vi "Node Example.vi"() -> ()   [LabVIEW 2016, in "PXImc Custom Device Engine.lvlib" / "PXImc Router.lvlib"]
uses:
  Shared/PXImc Router/Controls/Node - Configuration.ctl
  Shared/PXImc Router/Controls/Table Index-Size.ctl
  <vilib>/Utility/error.llb/DialogType.ctl
  Shared/PXImc Router/VIs/Node/Node - Globals.vi
  PXImc Router.lvlib
  Shared/PXImc Router/PXImc Router.lvlib
panel:
  in  "stop":bool
  out "Writer Node 2":T1(graph)={"[0]"=11.0, "[1]"=12.0, "[2]"=13.0, "[3]"=14.0, "[4]"=15.0, "[5]"=0.0, "[6]"=0.0, "[7]"=0.0, "[8]"=0.0}
  out "Writer Node 1":T1(graph)={"[0]"=1.0, "[1]"=2.0, "[2]"=3.0, "[3]"=4.0, "[4]"=5.0, "[5]"=0.0, "[6]"=0.0, "[7]"=0.0, "[8]"=0.0}
  out "Reader Node 2":T1(graph)
  out "Reader Node 1":T1(graph)
  in  "Node 2 Configuration Properties":T2={"Resource Name"="PXIMC2", "Node ID"=0, "Node Reader Conn Id"=4, "Node Writer Conn Id"=3, "Node # Channels"=5, "Writing Segments"={"Index"=5, "Size"=5}, "Reading Segments"={"Index"=0, "Size"=5}, "Connection Timeout (s)"=60.0, "Readers Buffer Size"=250000, "Slave IP Address"=""}
  in  "Node Configuration Properties":T2={"Resource Name"="PXIMC2", "Node ID"=0, "Node Reader Conn Id"=2, "Node Writer Conn Id"=1, "Node # Channels"=5, "Writing Segments"={"Index"=0, "Size"=5}, "Reading Segments"={"Index"=0, "Size"=5}, "Connection Timeout (s)"=60.0, "Readers Buffer Size"=250000, "Slave IP Address"=""}
  # "Node 1"
  # "Node 2"
  # "Node 2 => Node 1"
  # "Node 1 => Node 2"
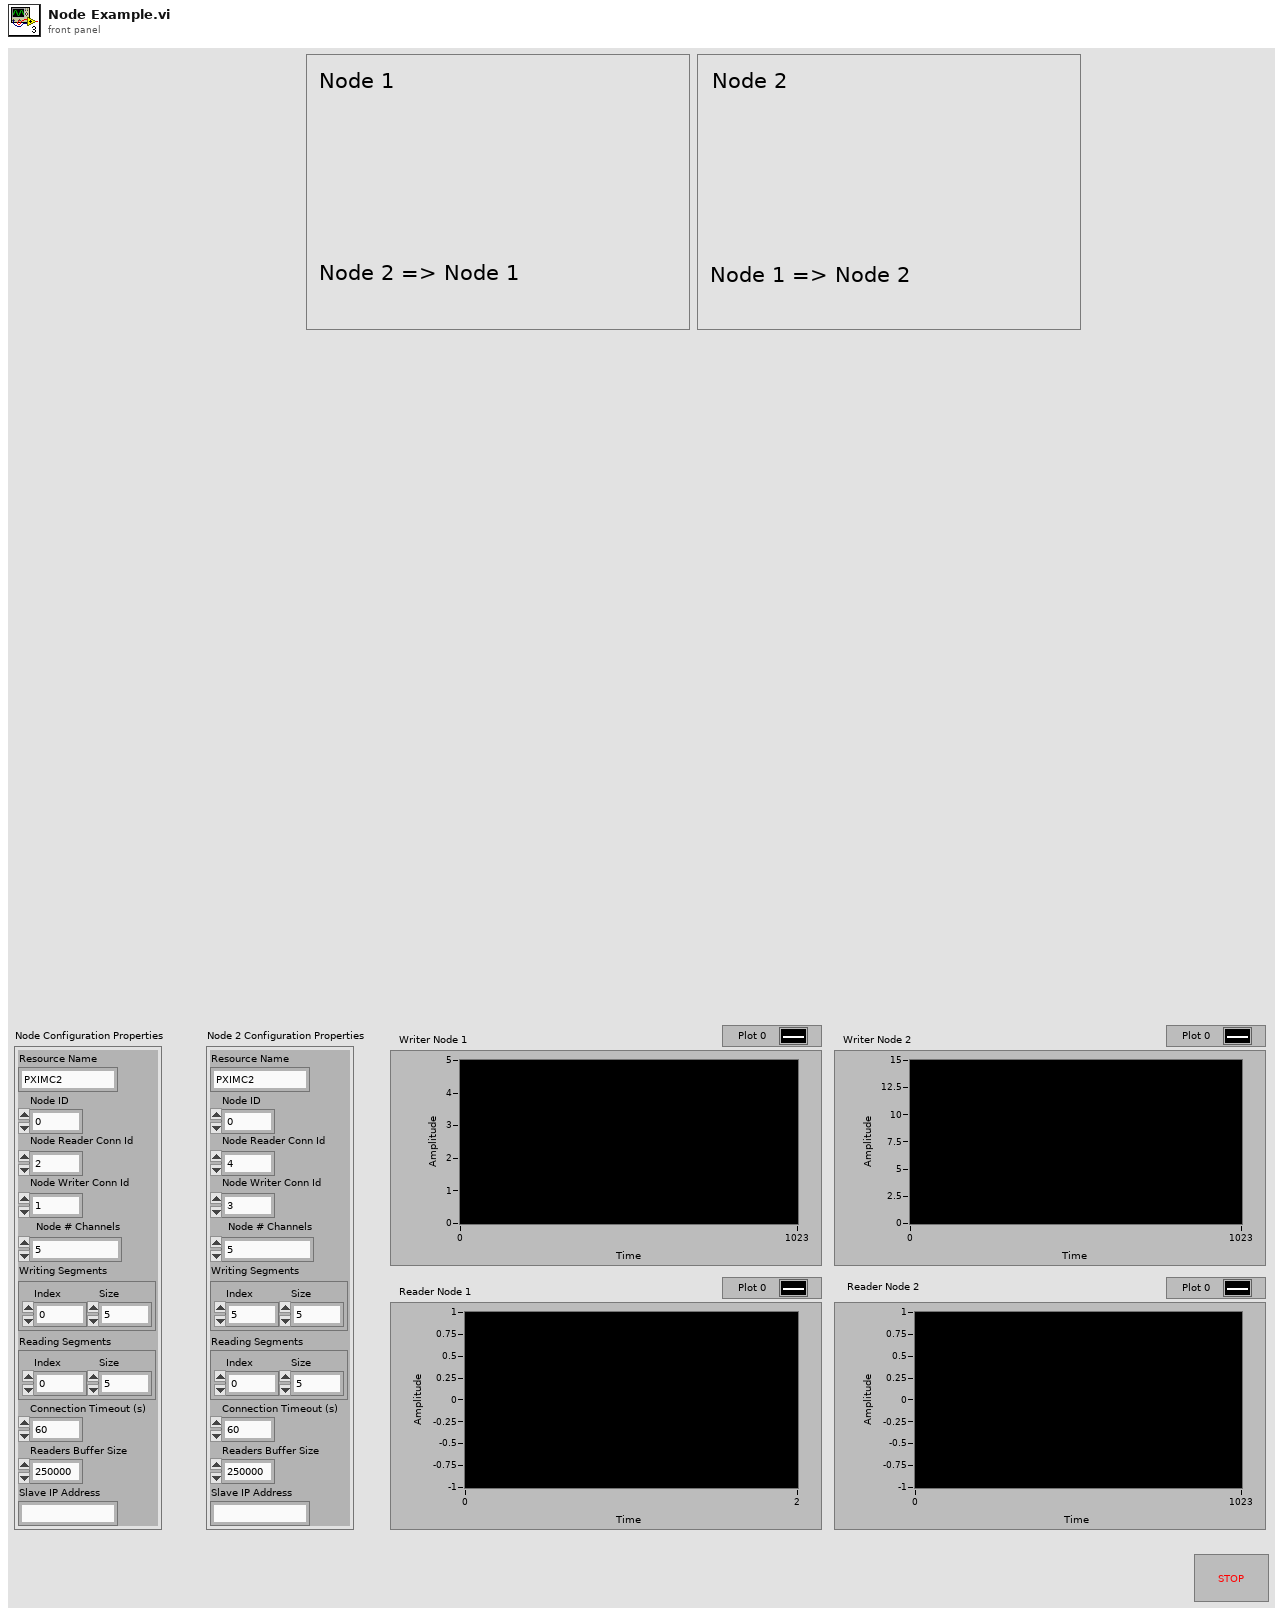
[diagram p1: front panel]
types:
  T1 = cluster{"[0]":dbl, "[1]":dbl, "[2]":dbl, "[3]":dbl, "[4]":dbl, "[5]":dbl, "[6]":dbl, "[7]":dbl, "[8]":dbl}
  T2 = typedef "PXImc Router.lvlib/Node - Configuration.ctl" = cluster{"Resource Name":string, "Node ID":u16, "Node Reader Conn Id":u16, "Node Writer Conn Id":u16, "Node # Channels":u32, "Writing Segments":T3, "Reading Segments":T3, "Connection Timeout (s)":dbl, "Readers Buffer Size":u32, "Slave IP Address":string}
  T3 = typedef "PXImc Router.lvlib/Table Index-Size.ctl" = cluster{"Index":u32, "Size":u32}
  T4 = typedef "DialogType.ctl" = u16
  T5 = typedef "PXImc Router.lvlib/Node Data.ctl" = cluster{"Writing Table":refnum<data-value>, "Reading Table":refnum<data-value>, "Reader Session":refnum<k21>, "Writer Session":refnum<k21>, "Reading Segment":T3, "Writing Segment":T3}
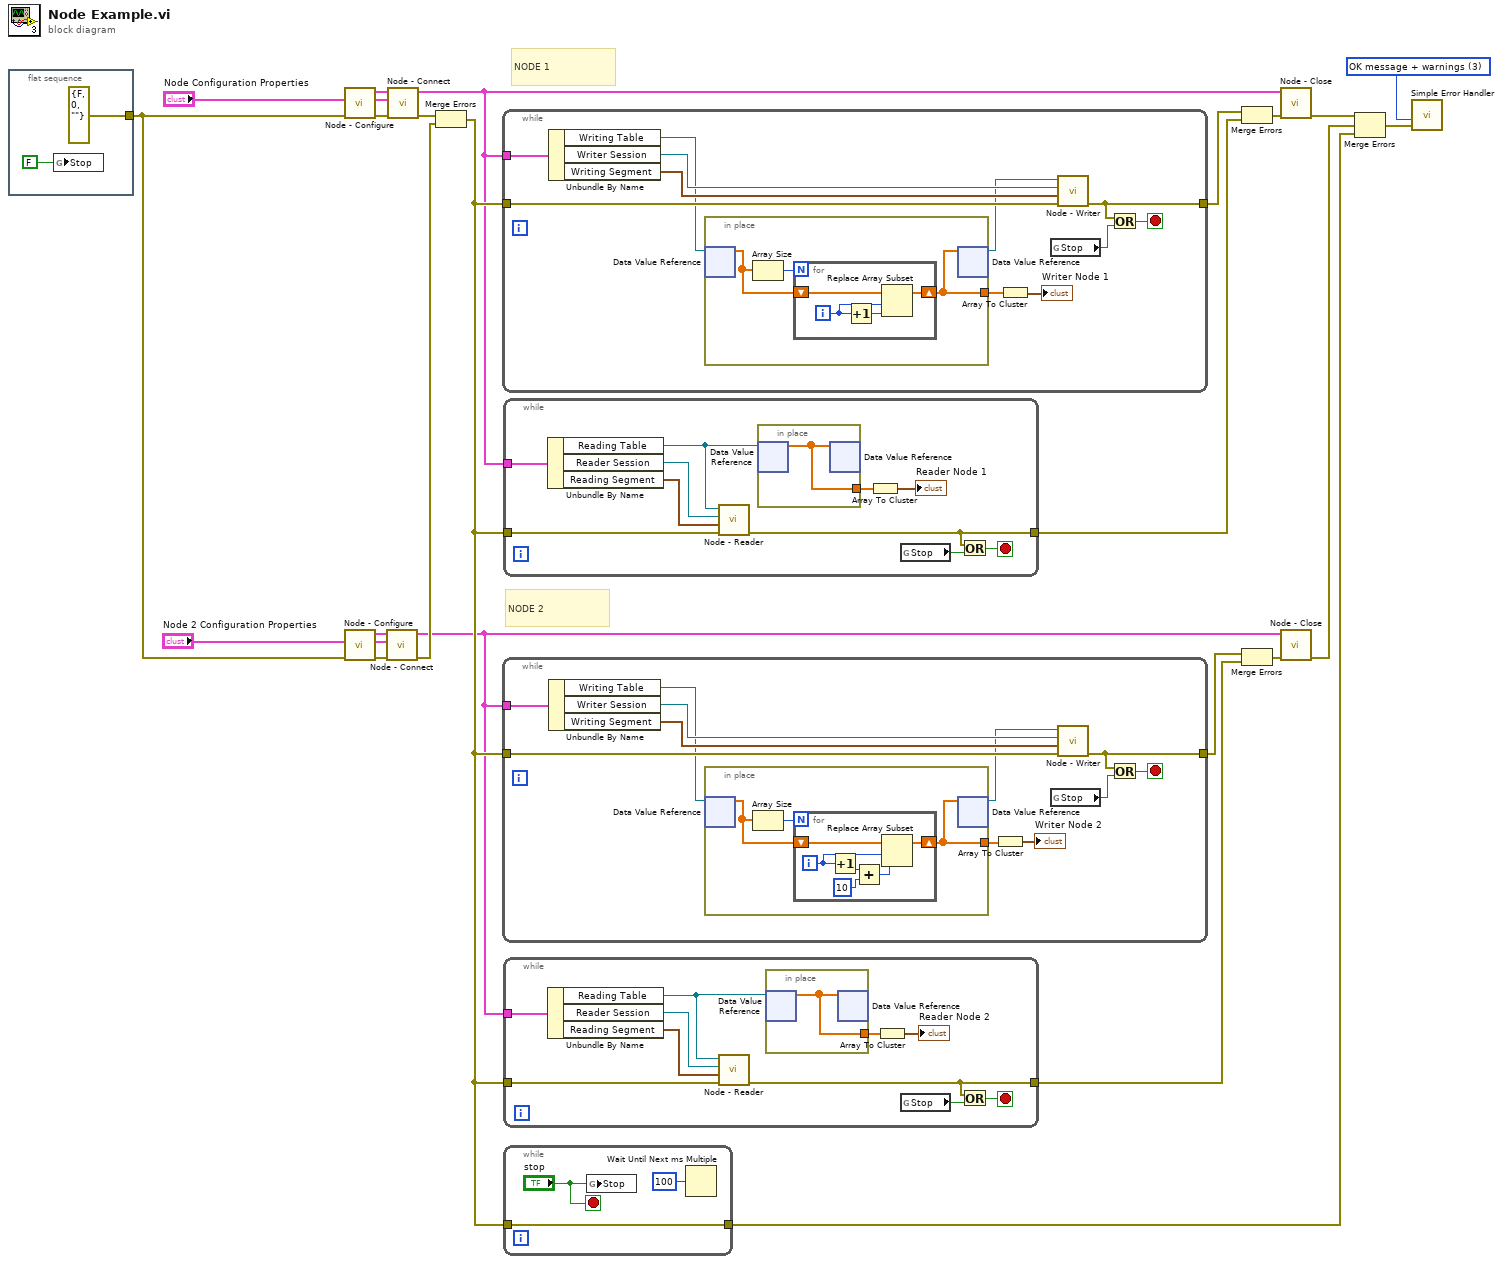
[diagram p0: block diagram]
diagram:
  w25 = T4 3 items=["no dialog", "OK message", "continue or stop message", "OK message + warnings", "continue/stop + warnings"] ("type of dialog (OK msg:1)")
  # "NODE 2"
  # "NODE 1"
  n1 = flat-sequence {
    tunnel: [errorcluster {"status"=FALSE, "code"=0, "source"=""} ("error constant")] -> w22
    frame #0 {
      n2 = global write "Node - Globals.vi" "Stop"(FALSE ("Stopped")) -> ()
    }
  }
  n3 = call "Node - Configure.vi"("error in (no error)"=w22, "Node Configuration Properties In"="Node Configuration Properties") -> ("error out"=w16:errorcluster, "Node Configuration Properties Out"=w17:T2, "Node Data"=w18:T5)  [unwired: 7 in]
  n4 = call "Node - Configure.vi"("error in (no error)"=w22, "Node Configuration Properties In"="Node 2 Configuration Properties") -> ("error out"=w12:errorcluster, "Node Configuration Properties Out"=w13:T2, "Node Data"=w14:T5)  [unwired: 7 in]
  n5 = call "Node - Connect.vi"("error in (no error)"=w12, "Configuration Properties In"=w13, "Node Data In"=w14) -> ("error out"=w11:errorcluster, "Node Data Out"=w7:T5)  [unwired: 6 in, 1 out]
  n6 = call "Node - Connect.vi"("error in (no error)"=w16, "Configuration Properties In"=w17, "Node Data In"=w18) -> ("error out"=w15:errorcluster, "Node Data Out"=w4:T5)  [unwired: 6 in, 1 out]
  n7 = Merge Errors(w15, w11) -> (w21:errorcluster)
  n8 = while {
    tunnel: w4 -> [w38]
    tunnel: w21 -> [w35]
    tunnel: [w30] -> w24
    stop <- w31 stop-if-true
    n9 = Unbundle By Name(w38) -> ("Writing Table"=w34:refnum<data-value>, "Writer Session"=w37:refnum<k21>, "Writing Segment"=w36:T3)
    n10 = in-place {
      in-place-border: [w39] -> w29
      n11 = in-place-dvr #1(w34) -> (w40:dbl[])  [unwired: 1 out]
      n12 = Array Size(array=w40) -> (size(s)=w41:i32)
      n13 = for {
        N: w41 -> [_]
        shift-right: [w44] -> w39
        shift-left: w40 -> [w45]
        i -> [w43]
        n14 = Increment(x=w43) -> (x+1=w42:i32)
        n15 = Replace Array Subset(array=w45, new element=w42, index=w43) -> (w44:dbl[])
      }
      n16 = in-place-dvr #1(w39) -> (w33:refnum<data-value>)  [unwired: 1 out]
    }
    n17 = Array To Cluster(array=w29) -> (cluster=→"Writer Node 1":T1)
    n18 = global read "Node - Globals.vi" "Stop"() -> (w32:bool)
    n19 = call "Node - Writer.vi"("error in (no error)"=w35, "Writing Segment"=w36, "PXImc Writing Session In"=w37, "Master Table Ref In"=w33) -> ("error out"=w30:errorcluster)  [unwired: 7 in]
    n20 = Or(x=w30, y=w32) -> (x .or. y?=w31:bool)
  }
  n21 = while {
    tunnel: w7 -> [w56]
    tunnel: w21 -> [w53]
    tunnel: [w48] -> w8
    stop <- w49 stop-if-true
    n22 = Unbundle By Name(w56) -> ("Writing Table"=w52:refnum<data-value>, "Writer Session"=w55:refnum<k21>, "Writing Segment"=w54:T3)
    n23 = in-place {
      in-place-border: [w57] -> w47
      n24 = in-place-dvr #2(w52) -> (w58:dbl[])  [unwired: 1 out]
      n25 = Array Size(array=w58) -> (size(s)=w59:i32)
      n26 = for {
        N: w59 -> [_]
        shift-right: [w64] -> w57
        shift-left: w58 -> [w65]
        i -> [w63]
        n27 = Increment(x=w63) -> (x+1=w62:i32)
        n28 = Add(x=w62, y=10) -> (x+y=w61:i32)
        n29 = Replace Array Subset(array=w65, new element=w61, index=w63) -> (w64:dbl[])
      }
      n30 = in-place-dvr #2(w57) -> (w51:refnum<data-value>)  [unwired: 1 out]
    }
    n31 = Array To Cluster(array=w47) -> (cluster=→"Writer Node 2":T1)
    n32 = global read "Node - Globals.vi" "Stop"() -> (w50:bool)
    n33 = call "Node - Writer.vi"("error in (no error)"=w53, "Writing Segment"=w54, "PXImc Writing Session In"=w55, "Master Table Ref In"=w51) -> ("error out"=w48:errorcluster)  [unwired: 7 in]
    n34 = Or(x=w48, y=w50) -> (x .or. y?=w49:bool)
  }
  n35 = while {
    tunnel: w4 -> [w75]
    tunnel: w21 -> [w74]
    tunnel: [w66] -> w23
    stop <- w71 stop-if-true
    n36 = Unbundle By Name(w75) -> ("Reading Table"=w70:refnum<data-value>, "Reader Session"=w73:refnum<k21>, "Reading Segment"=w67:T3)
    n37 = call "Node - Reader.vi"("error in (no error)"=w74, "Reading Segment"=w67, "PXImc Reading Session In"=w73, "Master Table Ref In"=w70) -> ("error out"=w66:errorcluster)  [unwired: 7 in]
    n38 = in-place {
      in-place-border: [w76] -> w69
      n39 = in-place-dvr #3(w70) -> (w76:dbl[])  [unwired: 1 out]
      n40 = in-place-dvr #3(w76) -> ()  [unwired: 2 out]
    }
    n41 = Array To Cluster(array=w69) -> (cluster=→"Reader Node 1":T1)
    n42 = global read "Node - Globals.vi" "Stop"() -> (w72:bool)
    n43 = Or(x=w66, y=w72) -> (x .or. y?=w71:bool)
  }
  n44 = while {
    tunnel: w7 -> [w86]
    tunnel: w21 -> [w85]
    tunnel: [w77] -> w5
    stop <- w81 stop-if-true
    n45 = Unbundle By Name(w86) -> ("Reading Table"=w80:refnum<data-value>, "Reader Session"=w84:refnum<k21>, "Reading Segment"=w83:T3)
    n46 = call "Node - Reader.vi"("error in (no error)"=w85, "Reading Segment"=w83, "PXImc Reading Session In"=w84, "Master Table Ref In"=w80) -> ("error out"=w77:errorcluster)  [unwired: 7 in]
    n47 = in-place {
      in-place-border: [w87] -> w79
      n48 = in-place-dvr #4(w80) -> (w87:dbl[])  [unwired: 1 out]
      n49 = in-place-dvr #4(w87) -> ()  [unwired: 2 out]
    }
    n50 = Array To Cluster(array=w79) -> (cluster=→"Reader Node 2":T1)
    n51 = global read "Node - Globals.vi" "Stop"() -> (w82:bool)
    n52 = Or(x=w77, y=w82) -> (x .or. y?=w81:bool)
  }
  n53 = while {
    tunnel: w21 -> [w89]
    tunnel: [w89] -> w2
    stop <- "stop" stop-if-true
    n54 = global write "Node - Globals.vi" "Stop"("stop") -> ()
    n55 = Wait Until Next ms Multiple(millisecond multiple=u32 100) -> ()  [unwired: 1 out]
  }
  n56 = Merge Errors(w24, w23) -> (w10:errorcluster)
  n57 = Merge Errors(w8, w5) -> (w6:errorcluster)
  n58 = call "Node - Close.vi"("error in (no error)"=w10, "Node Data In"=w4) -> ("error out"=w9:errorcluster)  [unwired: 9 in]
  n59 = call "Node - Close.vi"("error in (no error)"=w6, "Node Data In"=w7) -> ("error out"=w3:errorcluster)  [unwired: 9 in]
  n60 = Merge Errors(w9, w3, w2) -> (w1:errorcluster)
  n61 = call <vilib>:"Simple Error Handler.vi"("type of dialog (OK msg:1)"=w25, "error in (no error)"=w1) -> ()  [unwired: 3 in, 5 out]
